vi "Remove State.vi"(8 "Error In":errorcluster, 10 "State":string, 11 "UIM In":refnum<data-value>) -> (0 "Error Out":errorcluster, 3 "UIM Out":refnum<data-value>)   [LabVIEW 2015, in "UIM.lvclass"]
doc: "Remove the UI state previously saved in the UIM. If the state is not found, nothing happens."
uses:
  UIM.lvclass
  UIM.lvclass/UIM.ctl
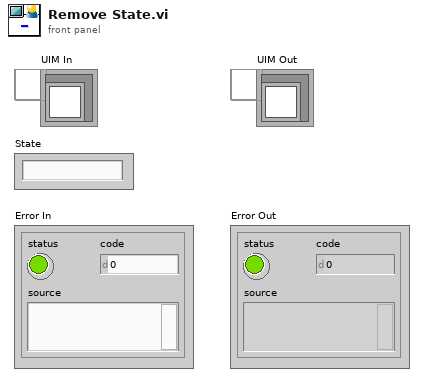
[diagram p1: front panel]
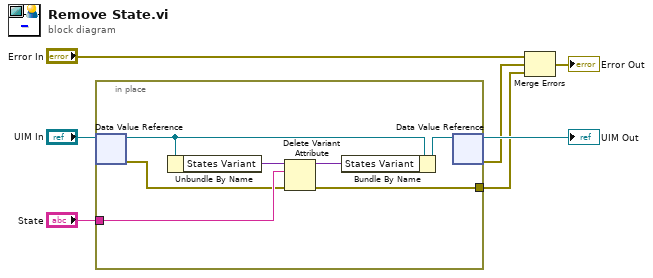
[diagram p0: block diagram]
diagram:
  n1 = in-place {
    in-place-border: [w8] -> w2
    in-place-border: "State" -> [w12]
    n2 = in-place-dvr #1("UIM In") -> (w14:refnum<class "UIM.lvclass">, w11:errorcluster)
    n3 = Unbundle By Name(w14) -> ("States Variant"=w13:variant)
    n4 = Delete Variant Attribute(4:w11, 6:w12, 7:w13) -> (0:w8:errorcluster, 3:w9:variant)  [unwired: 1 out]
    n5 = Bundle By Name(cluster=w14, "States Variant"=w9) -> (w10:refnum<class "UIM.lvclass">)
    n6 = in-place-dvr #1(w10) -> (→"UIM Out":refnum<data-value>, w1:errorcluster)
  }
  n7 = Merge Errors("Error In", w1, w2) -> (→"Error Out":errorcluster)
